vi "String.Check if is Match.vi"(7 "And(F)/Or(T)":bool, 10 "CSV Pattern List":string, 11 "String":string) -> (3 "Is Match":bool)   [LabVIEW 2024]
panel:
  out "Compare":bool[](array[boolean])
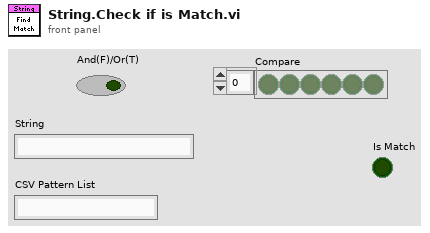
[diagram p1: front panel]
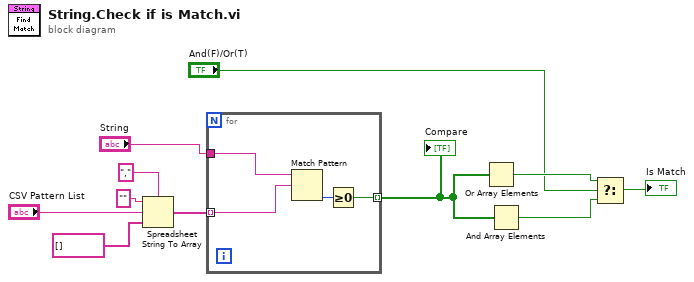
[diagram p0: block diagram]
diagram:
  n1 = Spreadsheet String To Array(delimiter (Tab)=",", format string="", spreadsheet string="CSV Pattern List", array type (2D Dbl)=string[] []) -> (array=w7:string[])
  n2 = for {
    tunnel: w7 -> [w13] mode=indexing
    tunnel: "String" -> [w14]
    tunnel: [w12] -> w5 mode=indexing
    n3 = Match Pattern(string=w14, regular expression=w13) -> (offset past match=w15:i32)  [unwired: 1 in, 3 out]
    n4 = Greater Or Equal To 0?(x=w15) -> (x >= 0?=w12:bool)
  }
  "Compare" <- w5
  n5 = Or Array Elements(Boolean array=w5) -> (logical OR=w4:bool)
  n6 = And Array Elements(Boolean array=w5) -> (logical AND=w3:bool)
  n7 = Select(t=w4, s="And(F)/Or(T)", f=w3) -> (s? t:f=→"Is Match":bool)
